vi "rp_wspr_read_file.vi"() -> ()   [LabVIEW 2014]
panel:
  in  "Path to WSPR file":path
  out "WSPR data":string
  out "error out":errorcluster
  out "Raw Python String Output":string
  out "Standard Error":string
  out "Return Code":i32
  in  "Path to Python.exe":path
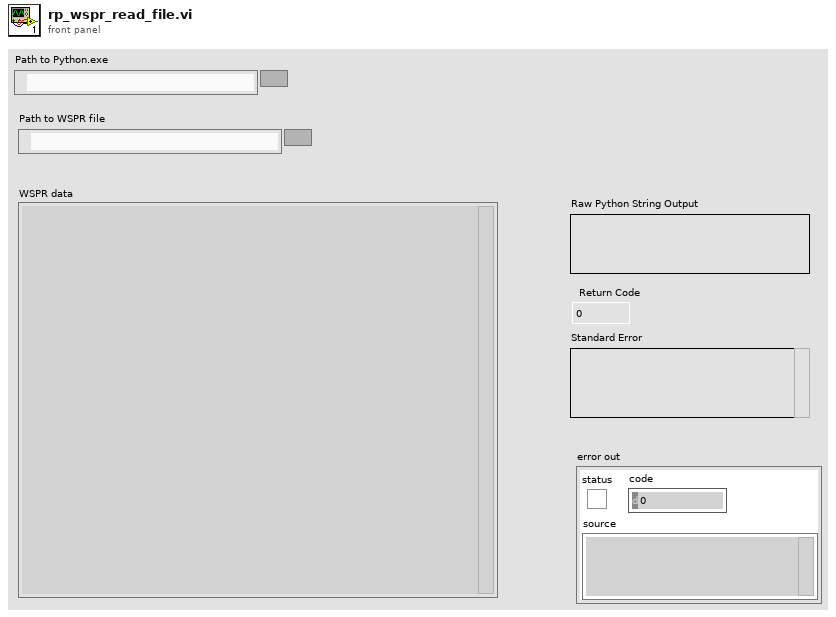
[diagram p1: front panel]
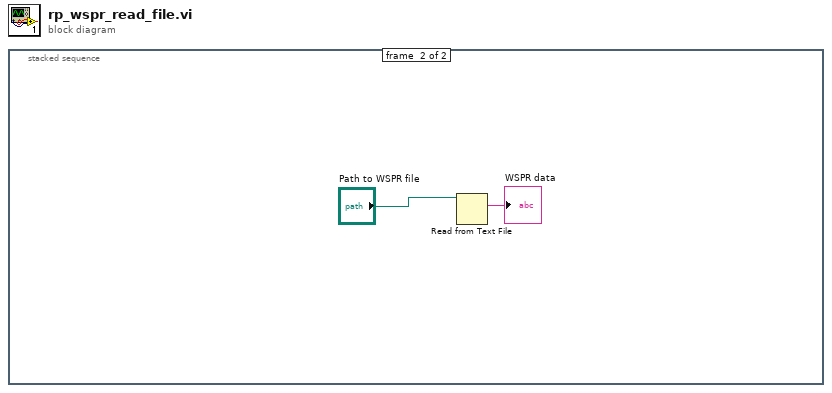
[diagram p0: block diagram]
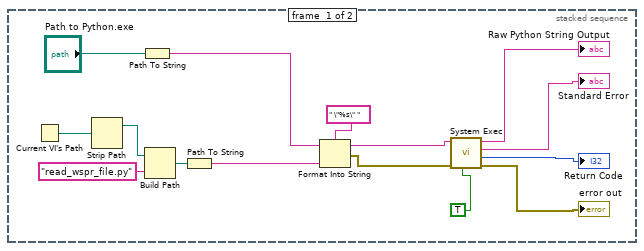
[diagram p2: hidden frame]
diagram:
  n1 = stacked-sequence {
    frame #0 {
      n2 = Current VI's Path() -> (path=w5:path)
      n3 = Strip Path(path=w5) -> (stripped path=w6:path)  [unwired: 1 out]
      n4 = Path To String(path="Path to Python.exe") -> (string=w15:string)
      n5 = Build Path(base path=w6, name or relative path="read_wspr_file.py" ("Path to Function")) -> (appended path=w3:path)
      n6 = Path To String(path=w3) -> (string=w2:string)
      n7 = Format Into String(format string=" \"%s\" ", initial string=w15, w2) -> (resulting string=w12:string, error out=w13:errorcluster)  [unwired: 1 in]
      n8 = call <vilib>:"System Exec.vi"("run minimized? (F)"=TRUE, "error in (no error)"=w13, "command line"=w12) -> ("error out"=→"error out":errorcluster, "return code"=→"Return Code":i32, "standard error"=→"Standard Error":string, "standard output"=→"Raw Python String Output":string)  [unwired: 5 in]
    }
    frame #1 {
      n9 = Read from Text File(file (use dialog)="Path to WSPR file") -> (text=→"WSPR data":string)  [unwired: 3 in, 3 out]
    }
  }
